vi "PTSequencer.ProcState.vi"(0 "i ref in":refnum<vi>, 2 "state timeout":i32=-1, 4 "state":string, 5 "error in":errorcluster) -> (14 "i ref out":refnum<vi>, 18 "next state":string, 19 "error out":errorcluster)   [LabVIEW 2014, in "PTSequencer.lvlib"]
uses:
  PTSequencer.lvlib
  CS_Core/CSSystem/CoreDefs/CoreDefs.error_type.ctl
  CS_Core/BaseSM/BaseSM.lvlib
  CS_Core/CSSystem/CoreLib/CoreLib.lvlib
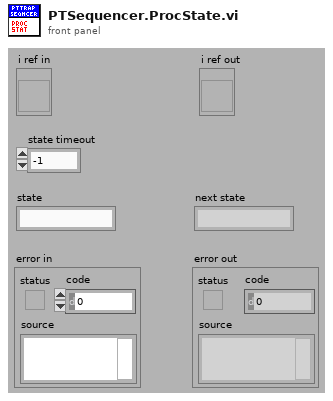
[diagram p1: front panel]
types:
  T1 = typedef "CoreDefs.error_type.ctl" = enum16{"no error", "can't load process", "can't unload process", "process does not exist", "can't install process", "can't remove process", "unknown function", "time out", "can't execute function", "duplicate queue name", "super not found", "caller queue invalid", "can't ping process", "unknown error", "VISA Error", "VISA timeout", "GPIB timeout", "GPIB error", "communication error", "data type mismatch", "can't read data from OPC server", "can't write data to OPC server", "OET error", "function not implemented", "process already exists", "invalid Shared Variable name", "error writing Shared Variable", "error reading Shared Variable", "invalid client name", "corrupt database", "unknown class", "call not authorized", "parameter out of range", "OET timeout: can't get data to modify", "invalid queue name", "requested operation incompatible with current state", "event undefined", "event disabled", "state undefined", "caller is not a friend", "EventBuilder: bad eventID", "EventBuilder: no DAQ devices", "a thread must not stop itself", "UNUSED ELEMENT4", "DiscArchiver: eventData incomplete", "DiscArchiver: eventData does not belong to run", "DiscArchiver: can't open file", "DiscArchiver: can't write to file", "DiscArchiver: available disc space low", "can't acquire semaphore", "error reading data from database", "notifier object is not existing", "can't register process", "can't unregister process", "illegal event type", "object disabled", "object already exists", "can't change state", "Instrument not found", "no connection to remote node", "invalid reference", "N/A", "UNUSED ELEMENT 1", "element not found", "illegal TCP/IP connection detected", "object does not exist", "invalid access ID", "unknown CS system", "invalid privilige", "unsupported data type", "unsupported server type", "IO server already exists", "Shared Variable already exists"}
  T2 = typedef "PTSequencer.lvlib/PTSequencer.i attribute.ctl" = cluster{"subsequence":bool, "mode":T3, "i step":i32, "nofLoops":i32, "i loop":i32, "Running":bool, "Paused":bool, "step done":bool, "loop done":bool, "seq done":bool, "DIM IDs":cluster{"step done":i32, "loop done":i32, "seq done":i32, "i step":i32, "i loop":i32}, "use stop conditions":bool, "stop conditions":T4[], "Step List":T6[], "DIM subsriptions":string[], "stop cond indexes":i32[], "step cond indexes":cluster{"step condition IDs":cluster{"step ID":i32, "condition ID":i32}[]}[], "Delay Start Time":timestamp, "status":string, "stopping":bool}
  T3 = typedef "PTSequencer.lvlib/PTSequencer.mode.ctl" = enum16{"single", "loop", "for loop"}
  T4 = typedef "PTSequencer.lvlib/PTSequencer.DIM service condition.ctl" = cluster{"DIM service":string, "descr":string, "nomValue":T5, "actValue":T5, "matched":bool, "DIM Status":cluster{"no link":bool, "quality":i32, "Time Stamp":timestamp}}
  T5 = typedef "CoreDefs.rawDataType.ctl" = i8[]
  T6 = typedef "PTSequencer.lvlib/PTSequencer.step.ctl" = cluster{"description":string, "object parameters":cluster{"object":string, "selector":string, "descriptor":string, "data":T5, "subsequence":bool, "call mode":enum16{"Simple DIM", "Synchronous"}, "data in":T5}, "result action":cluster{"check":bool, "passed":enum16{"Next", "Previous", "Repeat", "Jump"}, "failed":enum16{"Next", "Previous", "Repeat", "Jump"}, "jumpID_passed":i32, "jumpID_failed":i32}, "conditions":T4[], "fulfilled ":bool, "use delay":bool, "delay time (s)":dbl, "ID":i32}
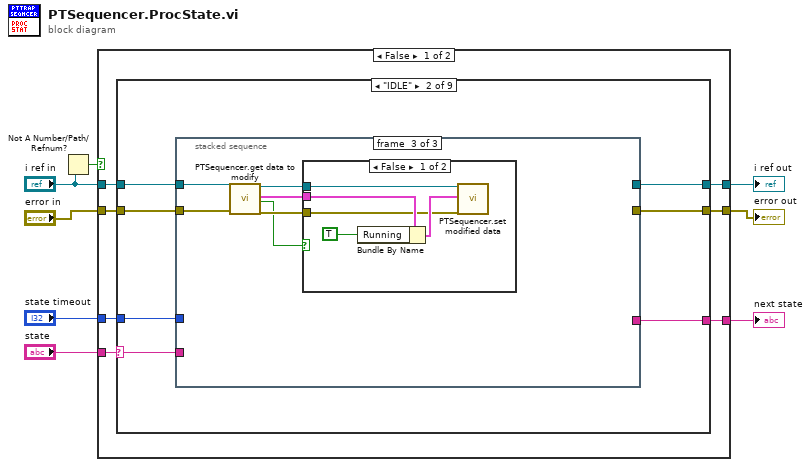
[diagram p0: block diagram]
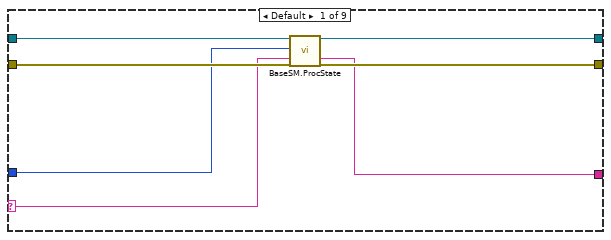
[diagram p2: hidden frame]
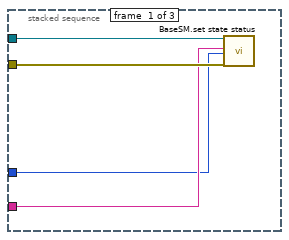
[diagram p3: hidden frame]
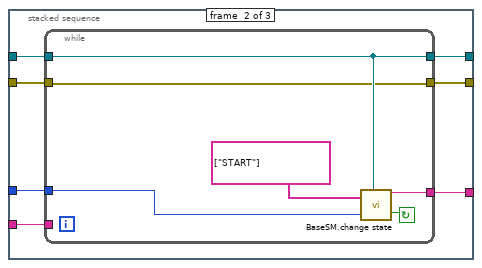
[diagram p4: hidden frame]
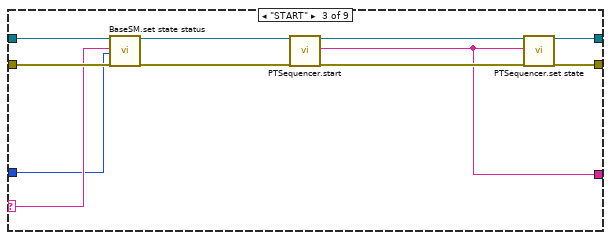
[diagram p6: hidden frame]
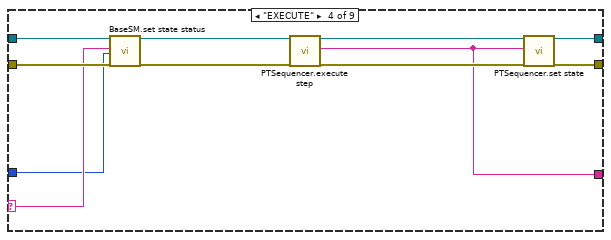
[diagram p7: hidden frame]
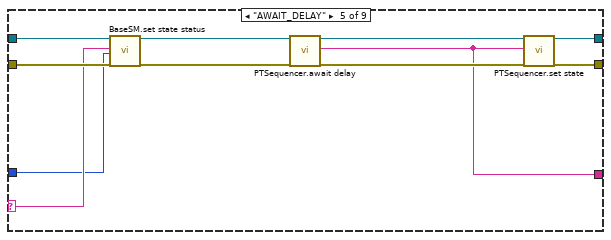
[diagram p8: hidden frame]
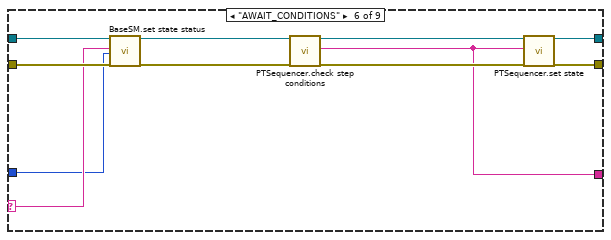
[diagram p9: hidden frame]
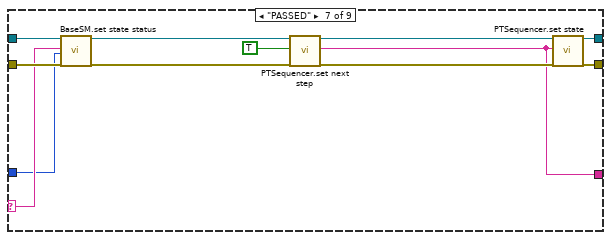
[diagram p10: hidden frame]
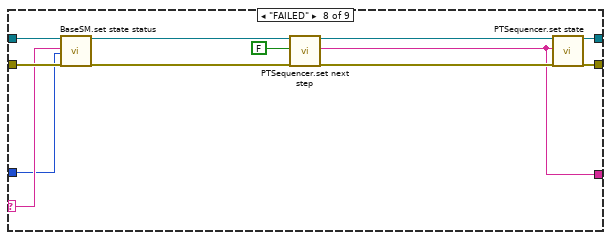
[diagram p11: hidden frame]
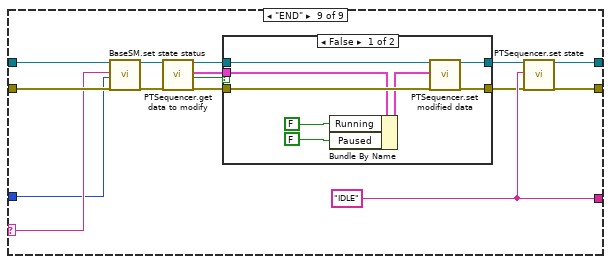
[diagram p12: hidden frame]
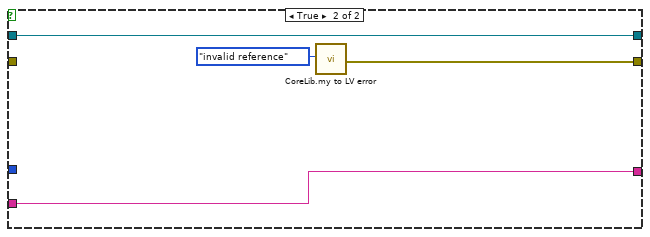
[diagram p14: hidden frame]
diagram:
  n1 = Not A Number/Path/Refnum?(number/path/refnum="i ref in") -> (NaN/Path/Refnum?=w2:bool)
  n2 = case shown="False" w2 {
    tunnel: "i ref in" -> [w15 w154]
    tunnel: [w14 w154] -> w8
    tunnel: "state" -> [w13 w151]
    tunnel: [w12 w151] -> w6
    tunnel: "state timeout" -> [w11 _]
    tunnel: "error in" -> [w10 _]
    tunnel: [w9 w152] -> w3
    frame False {
      n3 = case shown="\"IDLE\"" w13 {
        selector: w13 -> [w17 w26 w66 w77 w88 w99 w111 w123 w138]
        tunnel: w15 -> [w22 w29 w68 w79 w90 w101 w113 w125 w140]
        tunnel: [w21 w25 w64 w75 w86 w97 w109 w121 w136] -> w14
        tunnel: [w16 w23 w58 w69 w80 w91 w103 w115 w134] -> w12
        tunnel: w11 -> [w18 w27 w65 w76 w87 w98 w110 w122 w137]
        tunnel: w10 -> [w20 w28 w67 w78 w89 w100 w112 w124 w139]
        tunnel: [w19 w24 w63 w74 w85 w96 w108 w120 w135] -> w9
        frame Default {
          n4 = call "BaseSM.ProcState.vi"("i ref in"=w22, "state timeout [ms]"=w18, "state"=w17, "error in (no error)"=w20) -> ("i ref out"=w21:refnum<vi>, "next state"=w16:string, "error out"=w19:errorcluster)  [unwired: 13 in]
        }
        frame "IDLE" {
          n5 = stacked-sequence {
            tunnel: w26 -> [w31 w40 _]
            tunnel: [_ w39 _] -> w23
            tunnel: w29 -> [w33 w37 w52]
            tunnel: [_ w36 _] -> w25
            tunnel: w27 -> [w30 w38 _]
            tunnel: w28 -> [w32 w34 w51]
            tunnel: [_ w35 _] -> w24
            frame #0 {
              n6 = call "BaseSM.set state status.vi"("i ref in"=w33, "stateStatus"=w31, "ms timeout (10000)"=w30, "error in (no error)"=w32) -> ()  [unwired: 13 in, 3 out]
            }
            frame #1 {
              n7 = while {
                tunnel: w38 -> [w44]
                tunnel: [w46] -> w39
                tunnel: w40 -> [_]
                tunnel: w37 -> [w42]
                tunnel: [w42] -> w36
                tunnel: [w41] -> w35
                tunnel: w34 -> [w41]
                stop <- w45 continue-if-true
                n8 = call "BaseSM.change state.vi"("allowed next states"=string[] ["START"], "wait time [ms]"=w44, "i ref in"=w42) -> ("next state"=w46:string, "continue loop"=w45:bool)  [unwired: 13 in, 2 out]
              }
            }
            frame #2 {
              n9 = call "PTSequencer.get data to modify.vi"("i ref in"=w52, "error in (no error)"=w51) -> ("i ref out"=w50:refnum<vi>, "i attribute"=w49:T2, "timed out"=w47:bool, "error out"=w48:errorcluster)  [unwired: 14 in]
              n10 = case shown="False" w47 {
                tunnel: w50 -> [w57 _]
                tunnel: w49 -> [w56 _]
                tunnel: w48 -> [w53 _]
                frame False {
                  n11 = Bundle By Name(cluster=w56, "Running"=TRUE) -> (w55:T2)
                  n12 = call "PTSequencer.set modified data.vi"("i ref in"=w57, "CLASS.i attribute"=w55, "error in (no error)"=w53) -> ()  [unwired: 15 in, 2 out]
                }
                frame True {
                }
              }
            }
          }
        }
        frame "START" {
          n13 = call "BaseSM.set state status.vi"("i ref in"=w68, "stateStatus"=w66, "ms timeout (10000)"=w65, "error in (no error)"=w67) -> ("i ref out"=w62:refnum<vi>, "error out"=w61:errorcluster)  [unwired: 13 in, 1 out]
          n14 = call "PTSequencer.start.vi"("i ref in"=w62, "error in (no error)"=w61) -> ("i ref out"=w60:refnum<vi>, "next step"=w58:string, "error out"=w59:errorcluster)  [unwired: 14 in, 1 out]
          n15 = call "PTSequencer.set state.vi"("i ref in"=w60, "state"=w58, "error in (no error)"=w59) -> ("i ref out"=w64:refnum<vi>, "error out"=w63:errorcluster)  [unwired: 15 in]
        }
        frame "EXECUTE" {
          n16 = call "BaseSM.set state status.vi"("i ref in"=w79, "stateStatus"=w77, "ms timeout (10000)"=w76, "error in (no error)"=w78) -> ("i ref out"=w73:refnum<vi>, "error out"=w72:errorcluster)  [unwired: 13 in, 1 out]
          n17 = call "PTSequencer.execute step.vi"("i ref in"=w73, "error in (no error)"=w72) -> ("i ref out"=w71:refnum<vi>, "next step"=w69:string, "error out"=w70:errorcluster)  [unwired: 14 in, 1 out]
          n18 = call "PTSequencer.set state.vi"("i ref in"=w71, "state"=w69, "error in (no error)"=w70) -> ("i ref out"=w75:refnum<vi>, "error out"=w74:errorcluster)  [unwired: 15 in]
        }
        frame "AWAIT_DELAY" {
          n19 = call "BaseSM.set state status.vi"("i ref in"=w90, "stateStatus"=w88, "ms timeout (10000)"=w87, "error in (no error)"=w89) -> ("i ref out"=w84:refnum<vi>, "error out"=w83:errorcluster)  [unwired: 13 in, 1 out]
          n20 = call "PTSequencer.await delay.vi"("i ref in"=w84, "error in (no error)"=w83) -> ("i ref out"=w82:refnum<vi>, "next step"=w80:string, "error out"=w81:errorcluster)  [unwired: 15 in]
          n21 = call "PTSequencer.set state.vi"("i ref in"=w82, "state"=w80, "error in (no error)"=w81) -> ("i ref out"=w86:refnum<vi>, "error out"=w85:errorcluster)  [unwired: 15 in]
        }
        frame "AWAIT_CONDITIONS" {
          n22 = call "BaseSM.set state status.vi"("i ref in"=w101, "stateStatus"=w99, "ms timeout (10000)"=w98, "error in (no error)"=w100) -> ("i ref out"=w95:refnum<vi>, "error out"=w94:errorcluster)  [unwired: 13 in, 1 out]
          n23 = call "PTSequencer.check step conditions.vi"("i ref in"=w95, "error in (no error)"=w94) -> ("i ref out"=w93:refnum<vi>, "next state"=w91:string, "error out"=w92:errorcluster)  [unwired: 14 in, 1 out]
          n24 = call "PTSequencer.set state.vi"("i ref in"=w93, "state"=w91, "error in (no error)"=w92) -> ("i ref out"=w97:refnum<vi>, "error out"=w96:errorcluster)  [unwired: 15 in]
        }
        frame "PASSED" {
          n25 = call "BaseSM.set state status.vi"("i ref in"=w113, "stateStatus"=w111, "ms timeout (10000)"=w110, "error in (no error)"=w112) -> ("i ref out"=w107:refnum<vi>, "error out"=w106:errorcluster)  [unwired: 13 in, 1 out]
          n26 = call "PTSequencer.set next step.vi"("i ref in"=w107, "passed"=TRUE, "error in (no error)"=w106) -> ("i ref out"=w105:refnum<vi>, "next state"=w103:string, "error out"=w104:errorcluster)  [unwired: 13 in, 1 out]
          n27 = call "PTSequencer.set state.vi"("i ref in"=w105, "state"=w103, "error in (no error)"=w104) -> ("i ref out"=w109:refnum<vi>, "error out"=w108:errorcluster)  [unwired: 15 in]
        }
        frame "FAILED" {
          n28 = call "BaseSM.set state status.vi"("i ref in"=w125, "stateStatus"=w123, "ms timeout (10000)"=w122, "error in (no error)"=w124) -> ("i ref out"=w119:refnum<vi>, "error out"=w118:errorcluster)  [unwired: 13 in, 1 out]
          n29 = call "PTSequencer.set next step.vi"("i ref in"=w119, "passed"=FALSE, "error in (no error)"=w118) -> ("i ref out"=w117:refnum<vi>, "next state"=w115:string, "error out"=w116:errorcluster)  [unwired: 13 in, 1 out]
          n30 = call "PTSequencer.set state.vi"("i ref in"=w117, "state"=w115, "error in (no error)"=w116) -> ("i ref out"=w121:refnum<vi>, "error out"=w120:errorcluster)  [unwired: 15 in]
        }
        frame "END" {
          w134 = "IDLE"
          n31 = call "BaseSM.set state status.vi"("i ref in"=w140, "stateStatus"=w138, "ms timeout (10000)"=w137, "error in (no error)"=w139) -> ("i ref out"=w127:refnum<vi>, "error out"=w128:errorcluster)  [unwired: 13 in, 1 out]
          n32 = call "PTSequencer.get data to modify.vi"("i ref in"=w127, "error in (no error)"=w128) -> ("i ref out"=w131:refnum<vi>, "i attribute"=w133:T2, "timed out"=w132:bool, "error out"=w130:errorcluster)  [unwired: 14 in]
          n33 = case shown="False" w132 {
            tunnel: w130 -> [w148 w149]
            tunnel: w131 -> [w147 w150]
            tunnel: w133 -> [w146 _]
            tunnel: [w143 w150] -> w126
            tunnel: [w142 w149] -> w129
            frame False {
              n34 = Bundle By Name(cluster=w146, "Running"=FALSE ("Pause?"), "Paused"=FALSE ("Pause?")) -> (w144:T2)
              n35 = call "PTSequencer.set modified data.vi"("i ref in"=w147, "CLASS.i attribute"=w144, "error in (no error)"=w148) -> ("i ref out"=w143:refnum<vi>, "error out"=w142:errorcluster)  [unwired: 15 in]
            }
            frame True {
            }
          }
          n36 = call "PTSequencer.set state.vi"("i ref in"=w126, "state"=w134, "error in (no error)"=w129) -> ("i ref out"=w136:refnum<vi>, "error out"=w135:errorcluster)  [unwired: 15 in]
        }
      }
    }
    frame True {
      n37 = call "CoreLib.my to LV error.vi"("ErrorTypes"=CoreDefs.error_type."invalid reference") -> ("myErrorCluster"=w152:errorcluster)  [unwired: 17 in, 1 out]
    }
  }
  "i ref out" <- w8
  "next state" <- w6
  "error out" <- w3
